vi "write_peak_data.vi"(8 "error in (no error)":errorcluster caption="错误输入（无错误）", 10 "array in":dbl[](array[numeric]), 11 "refnum":T1 caption="引用句柄") -> (0 "error out":errorcluster caption="错误输出", 3 "refnum out":T1 caption="引用句柄输出")   [LabVIEW 2013]
uses:
  <vilib>/Utility/config.llb/Config Data RefNum.ctl
  <vilib>/Utility/config.llb/Write Key (Double).vi
  <vilib>/Utility/config.llb/NI_LVConfig.lvlib
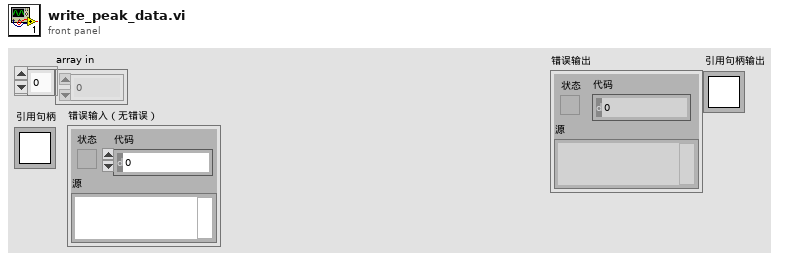
[diagram p1: front panel]
types:
  T1 = typedef "NI_LVConfig.lvlib/Config Data RefNum.ctl" = refnum<k1>
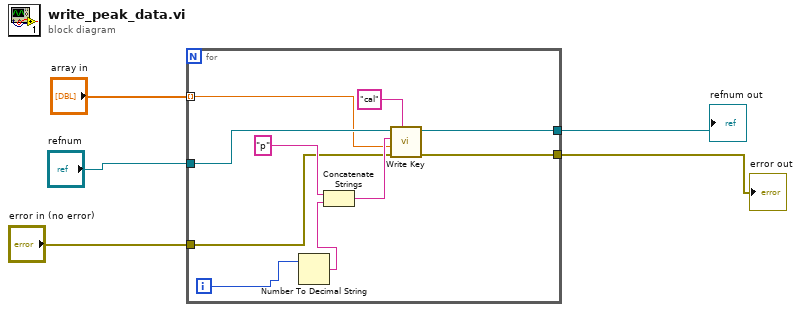
[diagram p0: block diagram]
diagram:
  n1 = for {
    tunnel: "array in" -> [w10] mode=indexing
    tunnel: "refnum" -> [w13]
    tunnel: "error in (no error)" -> [w9]
    tunnel: [w8] -> w2
    tunnel: [w7] -> w1
    i -> [w6]
    n2 = Number To Decimal String(number=w6) -> (decimal integer string=w14:string)  [unwired: 1 in]
    n3 = Concatenate Strings("p", w14) -> (w12:string)
    n4 = call-poly <vilib>:"Write Key.vi"("section"="cal", "error in (no error)"=w9, "value"=w10, "key"=w12, "refnum"=w13) -> ("error out"=w8:errorcluster, "refnum out"=w7:T1)  [unwired: 4 in, 1 out]
  }
  "error out" <- w2
  "refnum out" <- w1
